vi "WriteHeaders.vi"(8 "error in":errorcluster, 9 "Match Number":i32, 10 "Date and Time":string, 11 "File in":refnum<file>) -> (0 "error out":errorcluster, 3 "File out":refnum<file>)   [LabVIEW 2016]
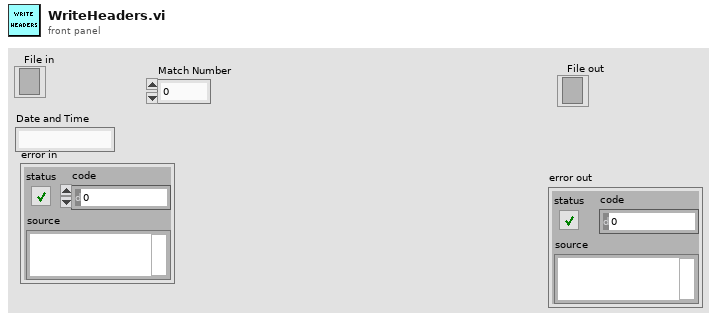
[diagram p1: front panel]
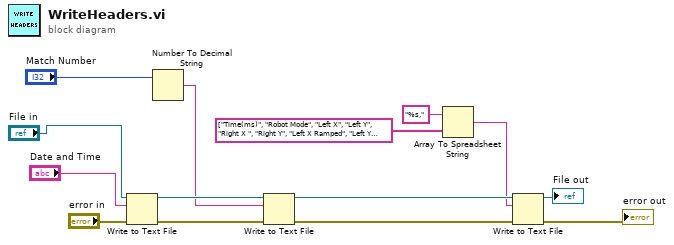
[diagram p0: block diagram]
diagram:
  n1 = Write to Text File(file (use dialog)="File in", text="Date and Time", error in="error in") -> (refnum out=w13:refnum<file>, error out=w14:errorcluster)  [unwired: 1 in, 1 out]
  n2 = Number To Decimal String(number="Match Number") -> (decimal integer string=w10:string)  [unwired: 1 in]
  n3 = Write to Text File(file (use dialog)=w13, text=w10, error in=w14) -> (refnum out=w6:refnum<file>, error out=w5:errorcluster)  [unwired: 1 in, 1 out]
  n4 = Array To Spreadsheet String(array=string[] ["Time(ms)", "Robot Mode", "Left X", "Left Y", "Right X ", "Right Y", "Left X Ramped", "Left Y Ramped", "Right X Ramped", "Right Y Ramped", "Diagnostic Messages", "Yaw", "Y axis acceleration", "Moving?", "Left Distance", "Right Distance", "Left Velocity", "Right Velocity", "Voltage", "Channel 0 current", "Channel 1 current", "Channel 2 current", "Channel 3 current", "Channel 4 current", "Channel 5 current", "Channel 6 current", "Channel 7 current", "Channel 8 current", "Channel 9 current"], 3:"%s," ("delimiter (Tab)")) -> (spreadsheet string=w4:string)  [unwired: 1 in]
  n5 = Write to Text File(file (use dialog)=w6, text=w4, error in=w5) -> (refnum out=→"File out":refnum<file>, error out=→"error out":errorcluster)  [unwired: 1 in, 1 out]
